vi "Rename.vi"(8 "error in (no error)":errorcluster, 10 "Name":string, 11 "FSM in":refnum<class "FSM.Node.lvclass">) -> (0 "error out":errorcluster, 3 "FSM out":refnum<class "FSM.Node.lvclass">)   [LabVIEW 2015, in "FSM.Node.lvclass"]
uses:
  FSM.Node.lvclass
  FSM.Node.lvclass/FSM.Node.ctl
  FSM.Port/FSM.Port.lvclass/FSM.Port.ctl
  FSM.Port/Write belongsTo.vi
  FSM.Port/FSM.Port.lvclass
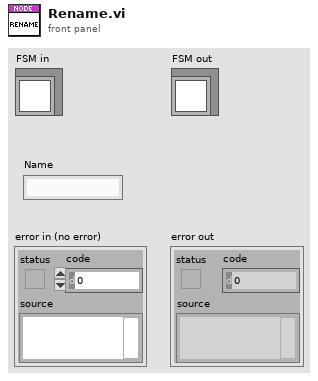
[diagram p1: front panel]
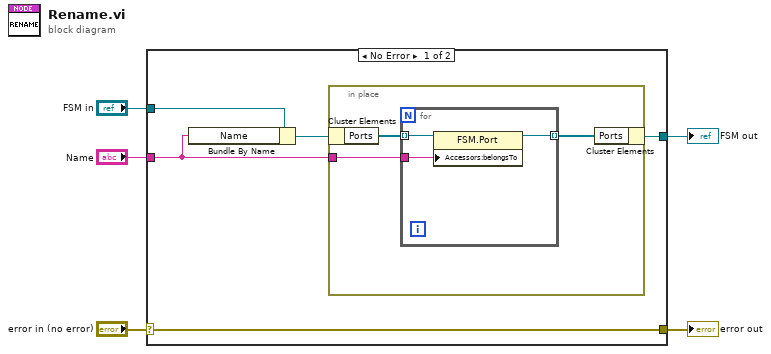
[diagram p0: block diagram]
diagram:
  n1 = case shown="No Error" "error in (no error)" {
    selector: "error in (no error)" -> [w9 w18]
    tunnel: [w9 w18] -> w4
    tunnel: [w7 w17] -> w2
    tunnel: "FSM in" -> [w10 w17]
    tunnel: "Name" -> [w6 _]
    frame No Error {
      n2 = Bundle By Name(cluster=w10, "Name"=w6) -> (w8:refnum<class "FSM.Node.lvclass">)
      n3 = in-place {
        in-place-border: w6 -> [w11]
        n4 = in-place-cluster #1(w8) -> ("Ports"=w13:refnum<class "FSM.Port.lvclass">[])
        n5 = for {
          tunnel: w13 -> [w16] mode=indexing
          tunnel: [w15] -> w12 mode=indexing
          tunnel: w11 -> [w14]
          n6 = property class="FSM.Port"(reference=w16, "Accessors:belongsTo"=w14) -> (reference out=w15:refnum<class "FSM.Port.lvclass">)  [unwired: 1 in, 1 out]
        }
        n7 = in-place-cluster #1("Ports"=w12) -> (w7:refnum<class "FSM.Node.lvclass">)
      }
    }
    frame Error {
    }
  }
  "error out" <- w4
  "FSM out" <- w2
